vi "Alarm logic.vi"(4 "124 lower mask":bool[](array[boolean])=[TRUE, TRUE, TRUE, TRUE, TRUE, TRUE, TRUE], 5 "124 upper mask":bool[](array[boolean])=[TRUE, TRUE, TRUE, TRUE, TRUE, TRUE, TRUE], 6 "Air Flow sw 2":bool, 7 "Air Flow sw 1":bool, 8 "294 mask":bool[](array[boolean])=[TRUE, TRUE, TRUE, TRUE, TRUE, TRUE, TRUE], 9 "Bldg 294 alarms":bool[](array[boolean]), 10 "Bldg 124 lower alarms":bool[](array[boolean]), 11 "Bldg 124 upper alarms":bool[](array[boolean])) -> (2 "Master Alarm 294":bool, 3 "Master Alarm  124":bool)   [LabVIEW 2012]
panel:
  # "Inputs: green - good, red - bad"
  # "124LL Fill Station"
  # "124UL Fill Station"
  # "100T Lab"
  # "Staff Lab"
  # "Cell 1"
  # "Cell 5"
  # "Cell 2"
  # "20T Lab"
  # "Cell 3"
  # "Laser Lab"
  # "Cell 4"
  # "Cell 6"
  # "PPMS Lab"
  # "Cave"
  # "(Any two bad O2) or (any one O2 and any one air flow) turn the alarm on"
  # "Any two bad turn the alarm on"
  # "60T Pit"
  # "100T Pit"
  # "294 Above Pits"
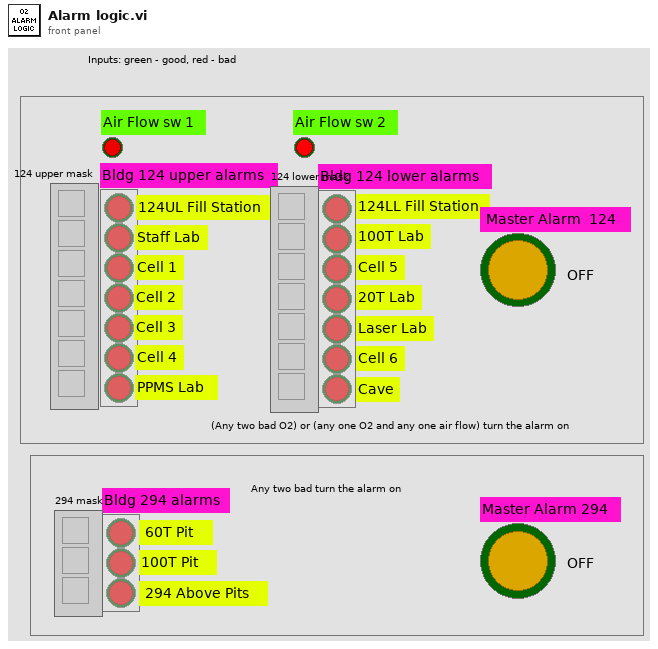
[diagram p1: front panel]
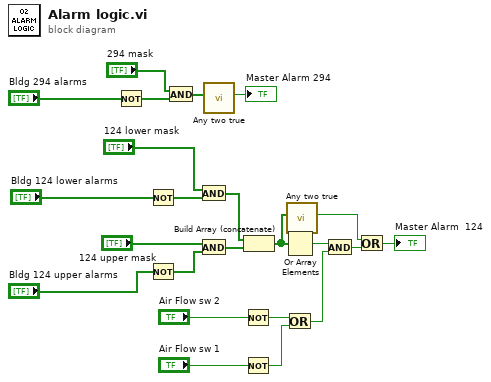
[diagram p0: block diagram]
diagram:
  n1 = Not(x="Bldg 294 alarms") -> (.not. x?=w8:bool[])
  n2 = Not(x="Bldg 124 lower alarms") -> (.not. x?=w11:bool[])
  n3 = Not(x="Bldg 124 upper alarms") -> (.not. x?=w1:bool[])
  n4 = And(x="294 mask", y=w8) -> (x .and. y?=w6:bool[])
  n5 = And(x="124 lower mask", y=w11) -> (x .and. y?=w5:bool[])
  n6 = And(x="124 upper mask", y=w1) -> (x .and. y?=w3:bool[])
  n7 = call "Any two true.vi"("Array in"=w6) -> ("Any two true?"=→"Master Alarm 294":bool)  [unwired: 10 in]
  n8 = Not(x="Air Flow sw 2") -> (.not. x?=w10:bool)
  n9 = Not(x="Air Flow sw 1") -> (.not. x?=w9:bool)
  n10 = Build Array (concatenate)(w5, w3) -> (w18:bool[])
  n11 = Or Array Elements(Boolean array=w18) -> (logical OR=w17:bool)
  n12 = Or(x=w10, y=w9) -> (x .or. y?=w16:bool)
  n13 = call "Any two true.vi"("Array in"=w18) -> ("Any two true?"=w14:bool)  [unwired: 10 in]
  n14 = And(x=w17, y=w16) -> (x .and. y?=w13:bool)
  n15 = Or(x=w14, y=w13) -> (x .or. y?=→"Master Alarm  124":bool)
